vi "Control - Set Settings.vi"(8 "error in (no error)":errorcluster, 11 "Folder Path":path) -> (0 "error out":errorcluster)   [LabVIEW 2017]
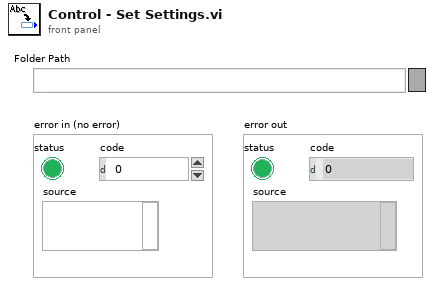
[diagram p1: front panel]
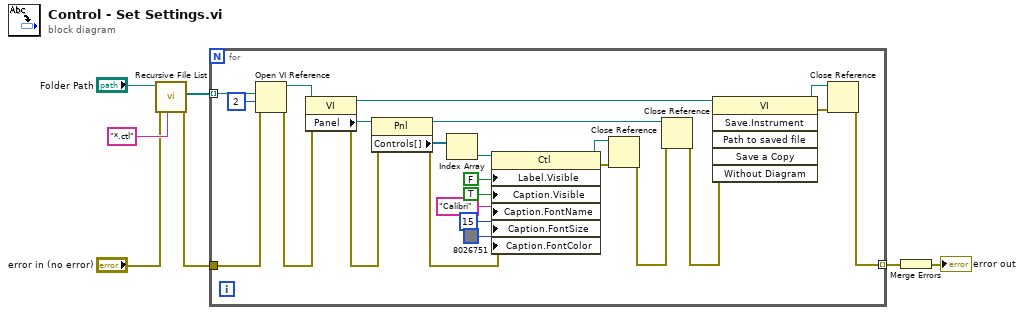
[diagram p0: block diagram]
diagram:
  n1 = call <vilib>:"Recursive File List.vi"("pattern"="*.ctl", "error in (no error)"="error in (no error)", "Folder Path"="Folder Path") -> ("error out"=w3:errorcluster, "All Files in Dir"=w4:path[])  [unwired: 4 in, 3 out]
  n2 = for {
    tunnel: w4 -> [w31] mode=indexing
    tunnel: w3 -> [w18]
    tunnel: [w8] -> w2 mode=indexing
    n3 = Open VI Reference(vi path=w31, options=2, error in (no error)=w18) -> (vi reference=w29:refnum<vi>, error out=w28:errorcluster)  [unwired: 3 in]
    n4 = property class="VI"(reference=w29, error in=w28) -> (reference out=w13:refnum<vi>, error out=w19:errorcluster, "Panel"=w27:refnum<vi>)
    n5 = property class="Pnl"(reference=w27, error in=w19) -> (reference out=w15:refnum<vi>, error out=w17:errorcluster, "Controls[]"=w26:refnum<vi>[])
    n6 = Index Array(array=w26) -> (element=w25:refnum<vi>)  [unwired: 1 in]
    n7 = property class="Ctl"(reference=w25, error in=w17, "Label.Visible"=FALSE, "Caption.Visible"=TRUE, "Caption.FontName"="Calibri" ("Font Name"), "Caption.FontSize"=u16 15 ("Size"), "Caption.FontColor"=u32 8026751 ("Color")) -> (reference out=w16:refnum<vi>, error out=w9:errorcluster)
    n8 = Close Reference(reference=w16, error in (no error)=w9) -> (error out=w14:errorcluster)
    n9 = Close Reference(reference=w15, error in (no error)=w14) -> (error out=w12:errorcluster)
    n10 = invoke class="VI" method="Save.Instrument"(reference=w13, error in=w12) -> (reference out=w11:refnum<vi>, error out=w10:errorcluster)  [unwired: 4 in, 4 out]
    n11 = Close Reference(reference=w11, error in (no error)=w10) -> (error out=w8:errorcluster)
  }
  n12 = Merge Errors(w2) -> (→"error out":errorcluster)
